vi "LEBITVacuum.ProcPeriodic.vi"(0 "i ref in":refnum<vi>, 3 "ms timeout (10000)":i32=10000, 5 "error in (no error)":errorcluster) -> (14 "i ref out":refnum<vi>, 17 "timed out":bool, 19 "error out":errorcluster)   [LabVIEW 2014, in "LEBITVacuum.lvlib"]
doc: "This method serves to periodically do things like reading values from the HW. Methods that should be executed periodically should be called from THIS methode. Add code here."
uses:
  LEBITVacuum.lvlib
  CSlibraries/UtilityLib/UtilityLib.valueStatus.ctl
  CSlibraries-extern/DimLVEvent/LVDimInterface/LVDimInterface.lvlib
  CS_Core/CSSystem/CoreLib/CoreLib.lvlib
  CSlibraries/UtilityLib/UtilityLib.lvlib
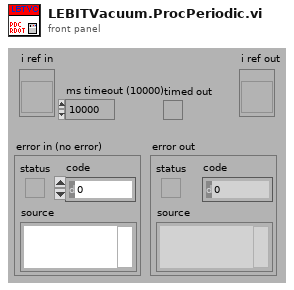
[diagram p1: front panel]
types:
  T1 = typedef "UtilityLib.lvlib/UtilityLib.valueStatus.ctl" = enum16{"no info available", "stand by/off", "on", "warning", "alarm/malfunction", "not implemented", "user action required", "important information", "system default", "control default", "indicator default", "button default"}
  T2 = typedef "LEBITVacuum.lvlib/LEBITVacuum.i attribute.ctl" = cluster{"setValuePLC":string[], "nickNames":string[], "setValuePLCServiceID":i32[], "monValuePLC":string[], "SetValueServiceID":i32[], "MonValueServiceID":i32[], "SetValue":i16[], "AllPLCValues":string[], "CondSpecial2DArray":string[][], "CondSpecialIndex":i32[], "ReasonForLocking":string, "ReasonForLockingID":i32, "enableValuePLC":string[], "OverwriteCloseSafetyPLC":string[], "OverwriteOpenSafetyPLC":string[], "OverwriteCloseSafetyPLCServiceID":i32[], "OverwriteOpenSafetyPLCServiceID":i32[], "MKS Address Array":i32[][], "MKS MeasurementServiceID":i32[], "MKS Measurement":string[], "CRYO Measurement":string[][], "CRYO MeasurementServiceID":i32[], "Special":string[], "Start Date":string, "MKS VISA resource":refnum<visa-resource-name>, "CRYO VISA resource":refnum<visa-resource-name>}
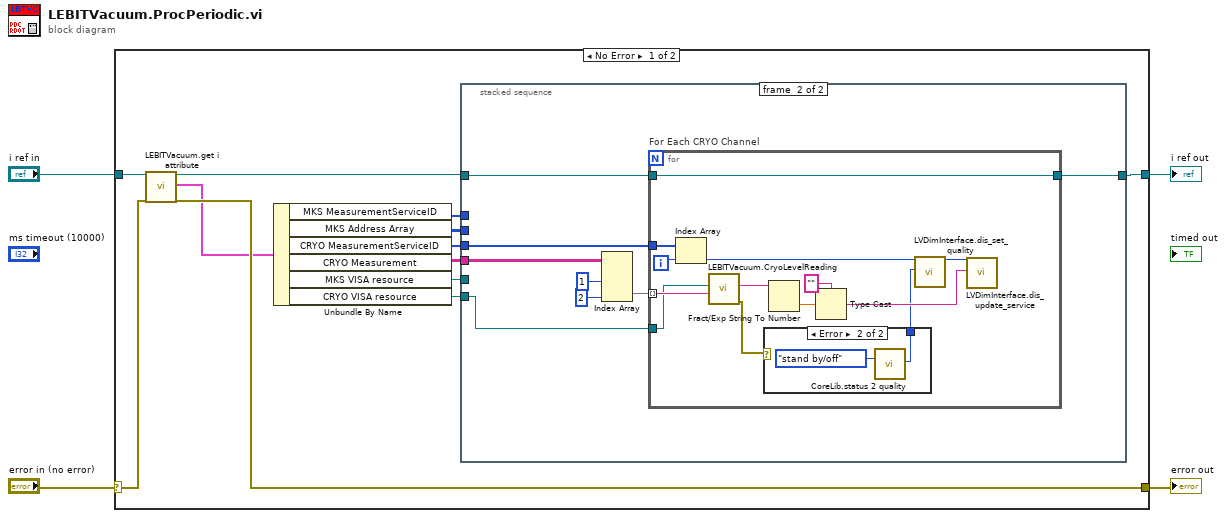
[diagram p0: block diagram]
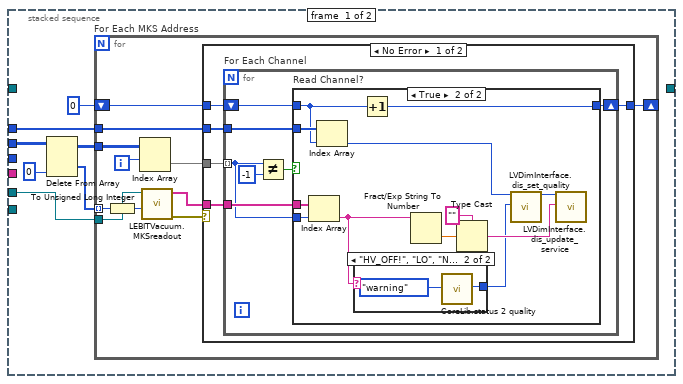
[diagram p2: hidden frame]
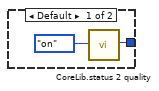
[diagram p4: hidden frame]
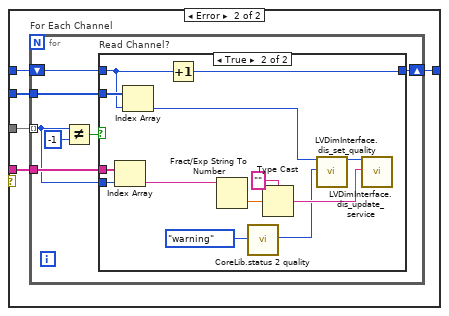
[diagram p5: hidden frame]
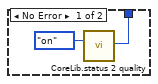
[diagram p7: hidden frame]
diagram:
  n1 = case shown="No Error" "error in (no error)" {
    selector: "error in (no error)" -> [w15 w115]
    tunnel: "i ref in" -> [w16 w116]
    tunnel: [w14 w116] -> w2
    tunnel: [w13 w115] -> w1
    frame No Error {
      n2 = call "LEBITVacuum.get i attribute.vi"("i ref in"=w16, "error in (no error)"=w15) -> ("i ref out"=w7:refnum<vi>, "i attribute"=w12:T2, "error out"=w13:errorcluster)  [unwired: 15 in]
      n3 = Unbundle By Name(w12) -> ("MKS MeasurementServiceID"=w10:i32[], "MKS Address Array"=w11:i32[][], "CRYO MeasurementServiceID"=w9:i32[], "CRYO Measurement"=w8:string[][], "MKS VISA resource"=w6:refnum<visa-resource-name>, "CRYO VISA resource"=w5:refnum<visa-resource-name>)
      n4 = stacked-sequence {
        tunnel: w11 -> [w23 _]
        tunnel: w10 -> [w20 _]
        tunnel: w7 -> [_ w97]
        tunnel: [_ w96] -> w14
        tunnel: w9 -> [_ w95]
        tunnel: w8 -> [_ w94]
        tunnel: w6 -> [w17 _]
        tunnel: w5 -> [_ w90]
        frame #0 {
          n5 = Delete From Array(array=w23, index (col)=0 ("disabled index (col)")) -> (deleted portion=w22:i32[], array with subset deleted=w21:i32[][])  [unwired: 2 in]
          n6 = for "For Each MKS Address" {
            tunnel: w22 -> [w34] mode=indexing
            tunnel: w21 -> [w33]
            tunnel: w20 -> [w30]
            shift-right: [w28] -> _
            shift-left: 0 -> [w29]
            tunnel: w17 -> [w25]
            i -> [w27]
            n7 = To Unsigned Long Integer(number=w34) -> (unsigned 32bit integer=w24:u32)
            n8 = Index Array(array=w33, index (row)=w27) -> (element=w32:i32[])  [unwired: 1 in]
            n9 = call "LEBITVacuum.MKSreadout.vi"("Binary Address"=w24, "Resource Name"=w25) -> ("error out"=w26:errorcluster, "Array"=w31:string[])  [unwired: 7 in]
            n10 = case shown="No Error" w26 {
              tunnel: w32 -> [w39 w68]
              tunnel: w31 -> [w38 w67]
              tunnel: w30 -> [w37 w66]
              tunnel: w29 -> [w36 w65]
              tunnel: [w35 w64] -> w28
              frame No Error {
                n11 = for "For Each Channel" {
                  tunnel: w39 -> [w40] mode=indexing
                  tunnel: w38 -> [w46]
                  tunnel: w37 -> [w45]
                  shift-right: [w44] -> w35
                  shift-left: w36 -> [w43]
                  n12 = Not Equal?(x=w40, y=-1) -> (x != y?=w41:bool)
                  n13 = case "Read Channel?" shown="True" w41 {
                    tunnel: w46 -> [_ w59]
                    tunnel: w45 -> [_ w55]
                    tunnel: [w47 w54] -> w44
                    tunnel: w43 -> [w47 w53]
                    tunnel: w40 -> [_ w52]
                    frame False {
                    }
                    frame True {
                      n14 = Index Array(array=w59, index=w52) -> (element=w48:string)
                      n15 = Index Array(array=w55, index=w53) -> (element=w50:i32)
                      n16 = case shown="\"HV_OFF!\", \"LO\", \"NOGAUGE!\"" w48 {
                        tunnel: [w61 w63] -> w51
                        frame Default {
                          n17 = call "CoreLib.status 2 quality.vi"("valueStatus"=UtilityLib.valueStatus."on") -> ("quality"=w61:i32)  [unwired: 18 in]
                        }
                        frame "HV_OFF!", "LO", "NOGAUGE!" {
                          n18 = call "CoreLib.status 2 quality.vi"("valueStatus"=UtilityLib.valueStatus."warning") -> ("quality"=w63:i32)  [unwired: 18 in]
                        }
                      }
                      n19 = Increment(x=w53) -> (x+1=w54:i32)
                      n20 = Fract/Exp String To Number(string=w48) -> (number=w57:dbl)  [unwired: 3 in, 1 out]
                      n21 = Type Cast(type="", x=w57) -> (*(type *) &x=w56:string)
                      n22 = call "LVDimInterface.dis_set_quality.vi"("my_serviceID"=w50, "quality"=w51) -> ("my_serviceID (out)"=w49:i32)  [unwired: 16 in, 1 out]
                      n23 = call "LVDimInterface.dis_update_service.vi"("my_serviceID"=w49, "data"=w56) -> ()  [unwired: 15 in, 3 out]
                    }
                  }
                }
              }
              frame Error {
                n24 = for "For Each Channel" {
                  tunnel: w68 -> [w69] mode=indexing
                  tunnel: w67 -> [w75]
                  tunnel: w66 -> [w74]
                  shift-right: [w73] -> w64
                  shift-left: w65 -> [w72]
                  n25 = Not Equal?(x=w69, y=-1) -> (x != y?=w70:bool)
                  n26 = case "Read Channel?" shown="True" w70 {
                    tunnel: w75 -> [_ w89]
                    tunnel: w74 -> [_ w85]
                    tunnel: [w76 w84] -> w73
                    tunnel: w72 -> [w76 w83]
                    tunnel: w69 -> [_ w82]
                    frame False {
                    }
                    frame True {
                      n27 = Index Array(array=w89, index=w82) -> (element=w78:string)
                      n28 = Index Array(array=w85, index=w83) -> (element=w80:i32)
                      n29 = Increment(x=w83) -> (x+1=w84:i32)
                      n30 = Fract/Exp String To Number(string=w78) -> (number=w87:dbl)  [unwired: 3 in, 1 out]
                      n31 = call "CoreLib.status 2 quality.vi"("valueStatus"=UtilityLib.valueStatus."warning") -> ("quality"=w81:i32)  [unwired: 18 in]
                      n32 = Type Cast(type="", x=w87) -> (*(type *) &x=w86:string)
                      n33 = call "LVDimInterface.dis_set_quality.vi"("my_serviceID"=w80, "quality"=w81) -> ("my_serviceID (out)"=w79:i32)  [unwired: 16 in, 1 out]
                      n34 = call "LVDimInterface.dis_update_service.vi"("my_serviceID"=w79, "data"=w86) -> ()  [unwired: 15 in, 3 out]
                    }
                  }
                }
              }
            }
          }
        }
        frame #1 {
          n35 = Index Array(array=w94, index (col) #1=1 ("index (row)"), index (col) #2=2 ("index (col)")) -> (element #2=w91:string[])  [unwired: 2 in, 1 out]
          n36 = for "For Each CRYO Channel" {
            tunnel: w95 -> [w109]
            tunnel: w97 -> [w110]
            tunnel: [w110] -> w96
            tunnel: w91 -> [w104] mode=indexing
            tunnel: w90 -> [w98]
            i -> [w103]
            n37 = Index Array(array=w109, index=w103) -> (element=w101:i32)
            n38 = call "LEBITVacuum.CryoLevelReading.vi"("Channels"=w104, "CRYO VISA resource"=w98) -> ("error out"=w99:errorcluster, "Data Out"=w105:string)  [unwired: 4 in]
            n39 = case shown="Error" w99 {
              tunnel: [w112 w114] -> w102
              frame No Error {
                n40 = call "CoreLib.status 2 quality.vi"("valueStatus"=UtilityLib.valueStatus."on") -> ("quality"=w112:i32)  [unwired: 18 in]
              }
              frame Error {
                n41 = call "CoreLib.status 2 quality.vi"("valueStatus"=UtilityLib.valueStatus."stand by/off") -> ("quality"=w114:i32)  [unwired: 18 in]
              }
            }
            n42 = Fract/Exp String To Number(string=w105) -> (number=w107:dbl)  [unwired: 3 in, 1 out]
            n43 = Type Cast(type="", x=w107) -> (*(type *) &x=w106:string)
            n44 = call "LVDimInterface.dis_set_quality.vi"("my_serviceID"=w101, "quality"=w102) -> ("my_serviceID (out)"=w100:i32)  [unwired: 16 in, 1 out]
            n45 = call "LVDimInterface.dis_update_service.vi"("my_serviceID"=w100, "data"=w106) -> ()  [unwired: 15 in, 3 out]
          }
        }
      }
    }
    frame Error {
    }
  }
  "error out" <- w1
  "i ref out" <- w2
